vi "OwningPane.vi"(6 "error in":errorcluster, 9 "Decoration in":refnum<class "Decoration.lvclass">) -> (0 "error out":errorcluster, 3 "Decoration out":refnum<class "Decoration.lvclass">, 4 "Owning Pane":i32)   [LabVIEW 2014, in "Decoration.lvclass"]
uses:
  Decoration.lvclass
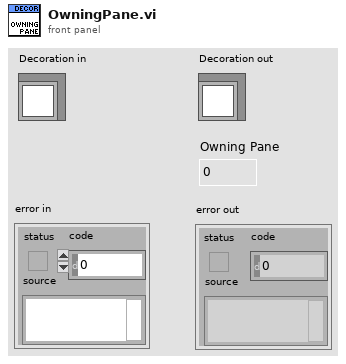
[diagram p1: front panel]
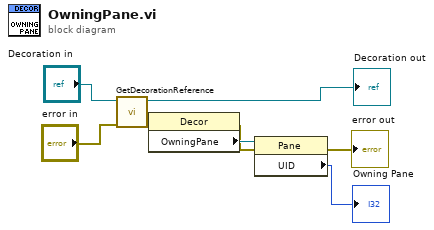
[diagram p0: block diagram]
diagram:
  n1 = call "GetDecorationReference.vi"("error in"="error in", "Decoration in"="Decoration in") -> ("error out"=w7:errorcluster, "Decoration reference"=w8:refnum<vi>, "Decoration out"=→"Decoration out":refnum<class "Decoration.lvclass">)  [unwired: 7 in]
  n2 = property class="Decor"(reference=w8, error in=w7) -> (error out=w4:errorcluster, "OwningPane"=w5:refnum<vi>)  [unwired: 1 out]
  n3 = property class="Pane"(reference=w5, error in=w4) -> (error out=→"error out":errorcluster, "UID"=→"Owning Pane":i32)  [unwired: 1 out]
